vi "Control Path.vi"(11 "DblControlEditorPanel in":refnum<class "DblControlEditorPanel.lvclass">) -> (2 "Control Path":path[](array[path]))   [LabVIEW 2020, in "VolatusGUIControls.lvlib" / "DblControlEditorPanel.lvclass"]
uses:
  DblControlEditorPanel.lvclass
  DblControlEditorPanel.lvclass/DblControlEditorPanel.ctl
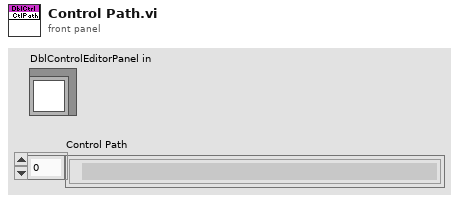
[diagram p1: front panel]
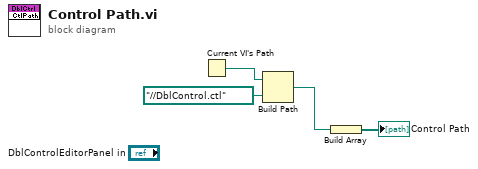
[diagram p0: block diagram]
diagram:
  n1 = Current VI's Path() -> (path=w4:path)
  n2 = Build Path(base path=w4, name or relative path=path "../../DblControl.ctl") -> (appended path=w2:path)
  n3 = Build Array(w2) -> (→"Control Path":path[])
